vi "Slave Property Node.vi"   [LabVIEW 2020]
doc: "Gets or reads properties of a Modbus slave. Use this node to read the daemon error and daemon status of a Modbus slave and to get the number of TCP connections and TCP connection information of a TCP Modbus slave. Daemon is a background process of Modbus slaves and responds to requests from Modbus master instances."
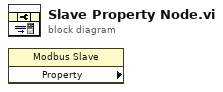
[diagram p0: block diagram]
diagram:
  n1 = property class="Modbus Slave" props=[]() -> ()  [unwired: 2 in, 3 out]
